vi "updateConfig.vi"(8 "error in":errorcluster, 11 "Config in":refnum<class "Config.lvclass">) -> (0 "error out":errorcluster, 3 "Config out":refnum<class "Config.lvclass">)   [LabVIEW 2020, in "Config.lvclass"]
uses:
  Config.lvclass
  Config.lvclass/Config.ctl
  <vilib>/Utility/config.llb/Read Key (String).vi
  <vilib>/Utility/config.llb/NI_LVConfig.lvlib
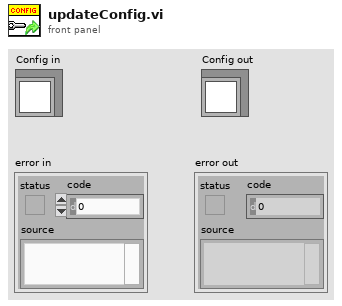
[diagram p1: front panel]
types:
  T1 = typedef "NI_LVConfig.lvlib/Config Data RefNum.ctl" = refnum<k1>
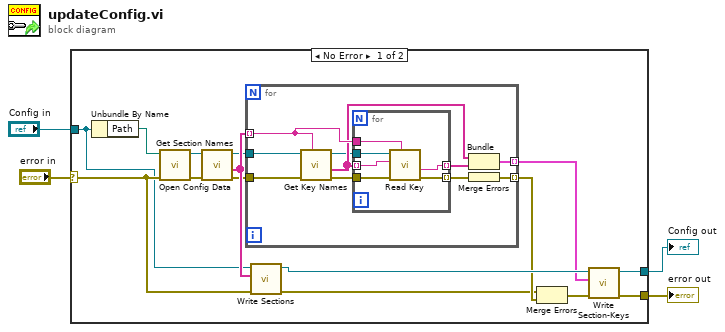
[diagram p0: block diagram]
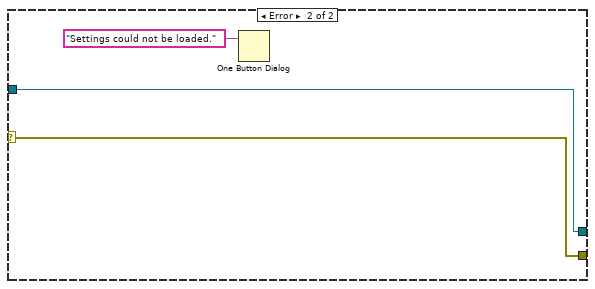
[diagram p2: hidden frame]
diagram:
  n1 = case shown="No Error" "error in" {
    selector: "error in" -> [w17 w38]
    tunnel: [w7 w38] -> w4
    tunnel: "Config in" -> [w5 w37]
    tunnel: [w12 w37] -> w2
    frame No Error {
      n2 = Unbundle By Name(w5) -> ("Path"=w6:path)
      n3 = call <vilib>:"Open Config Data.vi"("error in (no error)"=w17, "configuration file path"=w6) -> ("error out"=w18:errorcluster, "refnum"=w19:T1)  [unwired: 7 in, 1 out]
      n4 = call <vilib>:"Get Section Names.vi"("error in (no error)"=w18, "refnum"=w19) -> ("error out"=w14:errorcluster, "section names"=w16:string[], "refnum out"=w15:T1)  [unwired: 7 in]
      n5 = for {
        tunnel: w16 -> [w27] mode=indexing
        tunnel: w15 -> [w29]
        tunnel: w14 -> [w28]
        tunnel: [w24] -> w8 mode=indexing
        tunnel: [w21] -> w11 mode=indexing
        n6 = call <vilib>:"Get Key Names.vi"("section"=w27, "error in (no error)"=w28, "refnum"=w29) -> ("error out"=w23:errorcluster, "key names"=w26:string[], "refnum out"=w20:T1)  [unwired: 5 in, 1 out]
        n7 = for {
          tunnel: w26 -> [w35] mode=indexing
          tunnel: w27 -> [w34]
          tunnel: [w33] -> w25 mode=indexing
          tunnel: w23 -> [w32]
          tunnel: [w31] -> w22 mode=indexing
          tunnel: w20 -> [w30]
          n8 = call-poly <vilib>:"Read Key.vi"("section"=w34, "error in (no error)"=w32, "key"=w35, "refnum"=w30) -> ("error out"=w31:errorcluster, "value"=w33:string)  [unwired: 4 in, 2 out]
        }
        n9 = Bundle("key names"=w26, w25) -> (w24:cluster{"key names":string[], string[]})  [unwired: 1 in]
        n10 = Merge Errors(w22) -> (w21:errorcluster)
      }
      n11 = call "Write Sections.vi"("error in (no error)"=w17, "Sections"=w16, "Config in"=w5) -> ("error out"=w10:errorcluster, "Config out"=w13:refnum<class "Config.lvclass">)  [unwired: 7 in]
      n12 = Merge Errors(w10, w11) -> (w9:errorcluster)
      n13 = call "Write Section-Keys.vi"("error in (no error)"=w9, "Section-Keys"=w8, "Config in"=w13) -> ("error out"=w7:errorcluster, "Config out"=w12:refnum<class "Config.lvclass">)  [unwired: 7 in]
    }
    frame Error {
      n14 = One Button Dialog(message="Settings could not be loaded.") -> ()  [unwired: 1 in, 1 out]
    }
  }
  "error out" <- w4
  "Config out" <- w2
